vi "Export Database Changes to Text Files.vi"(10 "Database Changes":T1 {"Missing"."Node Ref" format="%.0x"; "Changed"."Old"."Node Ref" format="%.0x"}, 11 "Folder":path) -> (0 "error out":errorcluster)   [LabVIEW 2025, in "Protection and Counter Addon System Explorer.lvlib"]
uses:
  Protection and Counter Addon System Explorer.lvlib
  Types/Database Changes.ctl
  Types/Base Frame Info_NoVS.ctl
  Types/Base Frame Info.ctl
  <vilib>/NI VeriStand/Custom Device API/Custom Device Item Ref.ctl
  Types/Related CAN Frames.ctl
  Types/Related CAN Frames No VS.ctl
  <vilib>/Utility/error.llb/Trim Whitespace One-Sided.vi
  <vilib>/NI VeriStand/Custom Device API/Custom Device API.lvlib
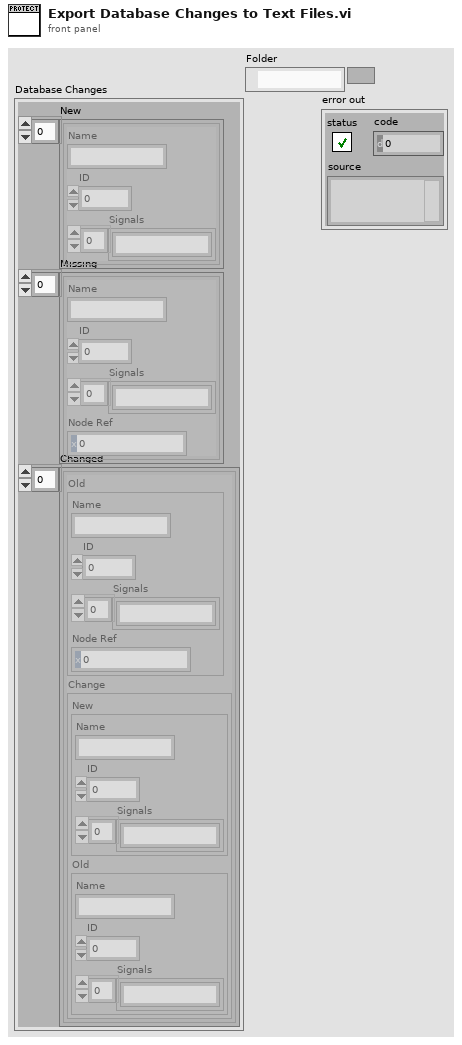
[diagram p1: front panel]
types:
  T1 = typedef "Protection and Counter Addon System Explorer.lvlib/Database Changes.ctl" = cluster{"New":T2[], "Missing":T3[], "Changed":T5[]}
  T2 = typedef "Protection and Counter Addon System Explorer.lvlib/Base Frame Info_NoVS.ctl" = cluster{"Name":string, "ID":u32, "Signals":string[]}
  T3 = typedef "Protection and Counter Addon System Explorer.lvlib/Base Frame Info.ctl" = cluster{"Name":string, "ID":u32, "Signals":string[], "Node Ref":T4}
  T4 = typedef "Custom Device API.lvlib/Custom Device Item Ref.ctl" = u64
  T5 = typedef "Protection and Counter Addon System Explorer.lvlib/Related CAN Frames.ctl" = cluster{"Old":T3, "Change":T6}
  T6 = typedef "Protection and Counter Addon System Explorer.lvlib/Related CAN Frames No VS.ctl" = cluster{"New":T2, "Old":T2}
  T7 = enum16{"open", "replace", "create", "open or create", "replace or create", "replace or create with confirmation"}
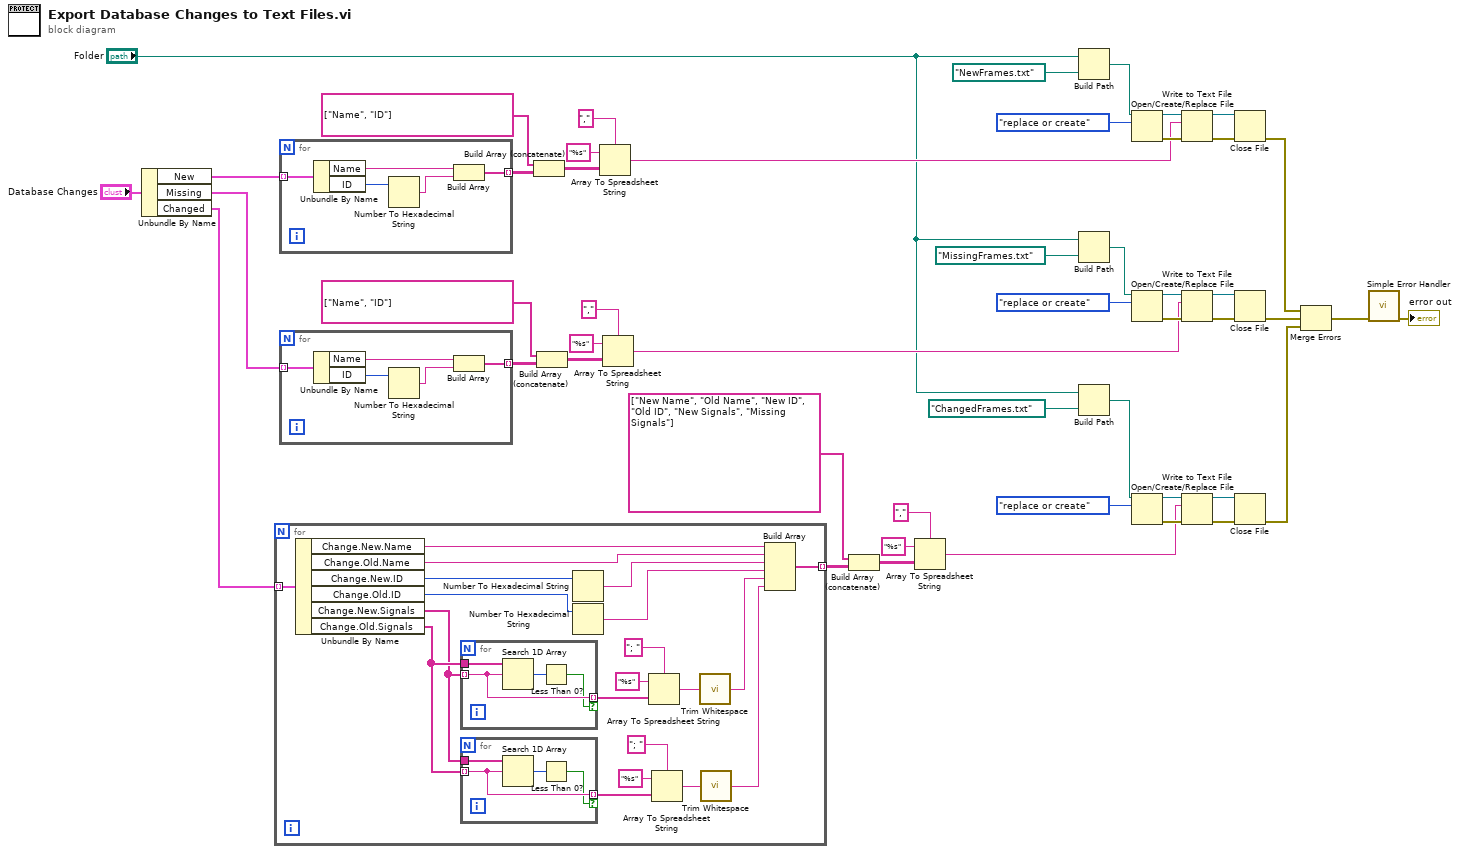
[diagram p0: block diagram]
diagram:
  n1 = Unbundle By Name("Database Changes") -> ("New"=w47:T2[], "Missing"=w48:T3[], "Changed"=w49:T5[])
  n2 = for {
    tunnel: w49 -> [w68] mode=indexing
    tunnel: [w62] -> w45 mode=indexing
    n3 = Unbundle By Name(w68) -> ("Change.New.Name"=w69:string, "Change.Old.Name"=w66:string, "Change.New.ID"=w67:u32, "Change.Old.ID"=w64:u32, "Change.New.Signals"=w60:string[], "Change.Old.Signals"=w61:string[])
    n4 = for {
      tunnel: w61 -> [w73]
      tunnel: w60 -> [w71] mode=indexing
      tunnel: [w71] -> w55 mode=indexing if=w70
      n5 = Search 1D Array(1D array=w73, element=w71) -> (index of element=w72:i32)  [unwired: 1 in]
      n6 = Less Than 0?(x=w72) -> (x < 0?=w70:bool)
    }
    n7 = for {
      tunnel: w60 -> [w77]
      tunnel: w61 -> [w75] mode=indexing
      tunnel: [w75] -> w58 mode=indexing if=w74
      n8 = Search 1D Array(1D array=w77, element=w75) -> (index of element=w76:i32)  [unwired: 1 in]
      n9 = Less Than 0?(x=w76) -> (x < 0?=w74:bool)
    }
    n10 = Number To Hexadecimal String(2:w67) -> (0:w65:string)  [unwired: 1 in]
    n11 = Number To Hexadecimal String(2:w64) -> (0:w63:string)  [unwired: 1 in]
    n12 = Array To Spreadsheet String(delimiter (Tab)="; ", array=w55, 3:"%s" ("format string")) -> (spreadsheet string=w54:string)
    n13 = Array To Spreadsheet String(delimiter (Tab)="; ", array=w58, 3:"%s" ("format string")) -> (spreadsheet string=w59:string)
    n14 = call <vilib>:"Trim Whitespace.vi"("string"=w54) -> ("trimmed string"=w51:string)  [unwired: 1 in]
    n15 = call <vilib>:"Trim Whitespace.vi"("string"=w59) -> ("trimmed string"=w50:string)  [unwired: 1 in]
    n16 = Build Array(w69, w66, w65, w63, w51, w50) -> (w62:string[])
  }
  n17 = for {
    tunnel: w47 -> [w82] mode=indexing
    tunnel: [w78] -> w37 mode=indexing
    n18 = Unbundle By Name(w82) -> ("Name"=w80:string, "ID"=w81:u32)
    n19 = Number To Hexadecimal String(2:w81) -> (0:w79:string)  [unwired: 1 in]
    n20 = Build Array(w80, w79) -> (w78:string[])
  }
  n21 = for {
    tunnel: w48 -> [w87] mode=indexing
    tunnel: [w83] -> w32 mode=indexing
    n22 = Unbundle By Name(w87) -> ("Name"=w85:string, "ID"=w86:u32)
    n23 = Number To Hexadecimal String(2:w86) -> (0:w84:string)  [unwired: 1 in]
    n24 = Build Array(w85, w84) -> (w83:string[])
  }
  n25 = Build Array (concatenate)(string[] ["Name", "ID"] ("appended array"), w37) -> (w40:string[][])
  n26 = Build Array (concatenate)(string[] ["Name", "ID"] ("appended array"), w32) -> (w35:string[][])
  n27 = Array To Spreadsheet String(delimiter (Tab)=",", array=w40, 3:"%s" ("format string")) -> (spreadsheet string=w25:string)
  n28 = Array To Spreadsheet String(delimiter (Tab)=",", array=w35, 3:"%s" ("format string")) -> (spreadsheet string=w19:string)
  n29 = Build Array (concatenate)(string[] ["New Name", "Old Name", "New ID", "Old ID", "New Signals", "Missing Signals"] ("appended array"), w45) -> (w43:string[][])
  n30 = Array To Spreadsheet String(delimiter (Tab)=",", array=w43, 3:"%s" ("format string")) -> (spreadsheet string=w13:string)
  n31 = Build Path(base path="Folder", name or relative path=path "NewFrames.txt") -> (appended path=w7:path)
  n32 = Build Path(base path="Folder", name or relative path=path "MissingFrames.txt") -> (appended path=w8:path)
  n33 = Build Path(base path="Folder", name or relative path=path "ChangedFrames.txt") -> (appended path=w9:path)
  n34 = Open/Create/Replace File(file path (use dialog)=w7, operation (0:open)=T7."replace or create") -> (refnum out=w29:refnum<file>, error out=w28:errorcluster)  [unwired: 4 in, 1 out]
  n35 = Open/Create/Replace File(file path (use dialog)=w8, operation (0:open)=T7."replace or create") -> (refnum out=w23:refnum<file>, error out=w22:errorcluster)  [unwired: 4 in, 1 out]
  n36 = Open/Create/Replace File(file path (use dialog)=w9, operation (0:open)=T7."replace or create") -> (refnum out=w17:refnum<file>, error out=w16:errorcluster)  [unwired: 4 in, 1 out]
  n37 = Write to Text File(file (use dialog)=w29, text=w25, error in=w28) -> (refnum out=w26:refnum<file>, error out=w27:errorcluster)  [unwired: 1 in, 1 out]
  n38 = Write to Text File(file (use dialog)=w23, text=w19, error in=w22) -> (refnum out=w20:refnum<file>, error out=w21:errorcluster)  [unwired: 1 in, 1 out]
  n39 = Write to Text File(file (use dialog)=w17, text=w13, error in=w16) -> (refnum out=w14:refnum<file>, error out=w15:errorcluster)  [unwired: 1 in, 1 out]
  n40 = Close File(refnum=w26, error in=w27) -> (error out=w5:errorcluster)  [unwired: 1 out]
  n41 = Close File(refnum=w20, error in=w21) -> (error out=w4:errorcluster)  [unwired: 1 out]
  n42 = Close File(refnum=w14, error in=w15) -> (error out=w3:errorcluster)  [unwired: 1 out]
  n43 = Merge Errors(w5, w4, w3) -> (w2:errorcluster)
  n44 = call <vilib>:"Simple Error Handler.vi"("error in (no error)"=w2) -> ("error out"=→"error out":errorcluster)  [unwired: 4 in, 4 out]
